vi "OLD Read Data File.vi"(0 "Filepath":path, 11 "Error In":errorcluster) -> (3 "Data":string[][](array[string]), 4 "Stats":string[][](array[string]), 6 "TestCfgCluster":T1, 8 "Serial Numbers":string[][](array[string]), 10 "TestParameters":string[][](array[string]), 15 "Error Out":errorcluster)   [LabVIEW 2013]
uses:
  TypeDef/TestCfgCluster.ctl
  TypeDef/Controller Names.ctl
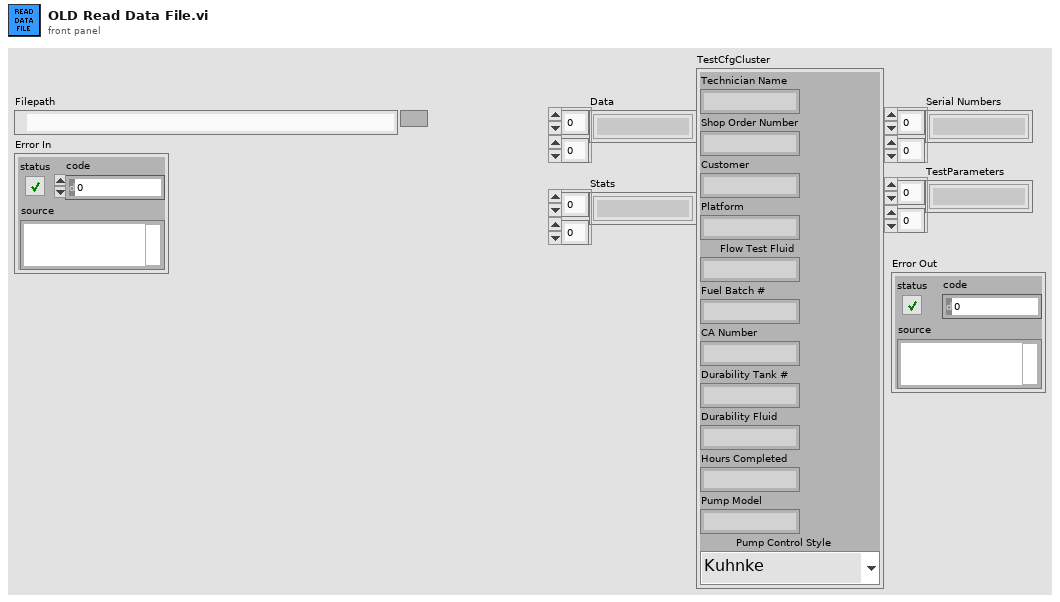
[diagram p1: front panel]
types:
  T1 = typedef "TestCfgCluster.ctl" = cluster{"Technician Name":string, "Shop Order Number":string, "Customer":string, "Platform":string, "Flow Test Fluid":string, "Fuel Batch #":string, "CA Number":string, "Durability Tank #":string, "Durability Fluid":string, "Hours Completed":string, "Pump Model":string, "Pump Control Style":T2}
  T2 = typedef "Controller Names.ctl" = enum16{"Kuhnke", "Conti", "Helbako", "TI PWM", "PSA", "Hella Gas", "Hella Diesel", "8 Comm", "10 Comm", "8 Comm Hella", "10 Comm Hella", "8 Comm Omron", "10 Comm Omron", "8 Comm Nissan", "10 Comm Nissan"}
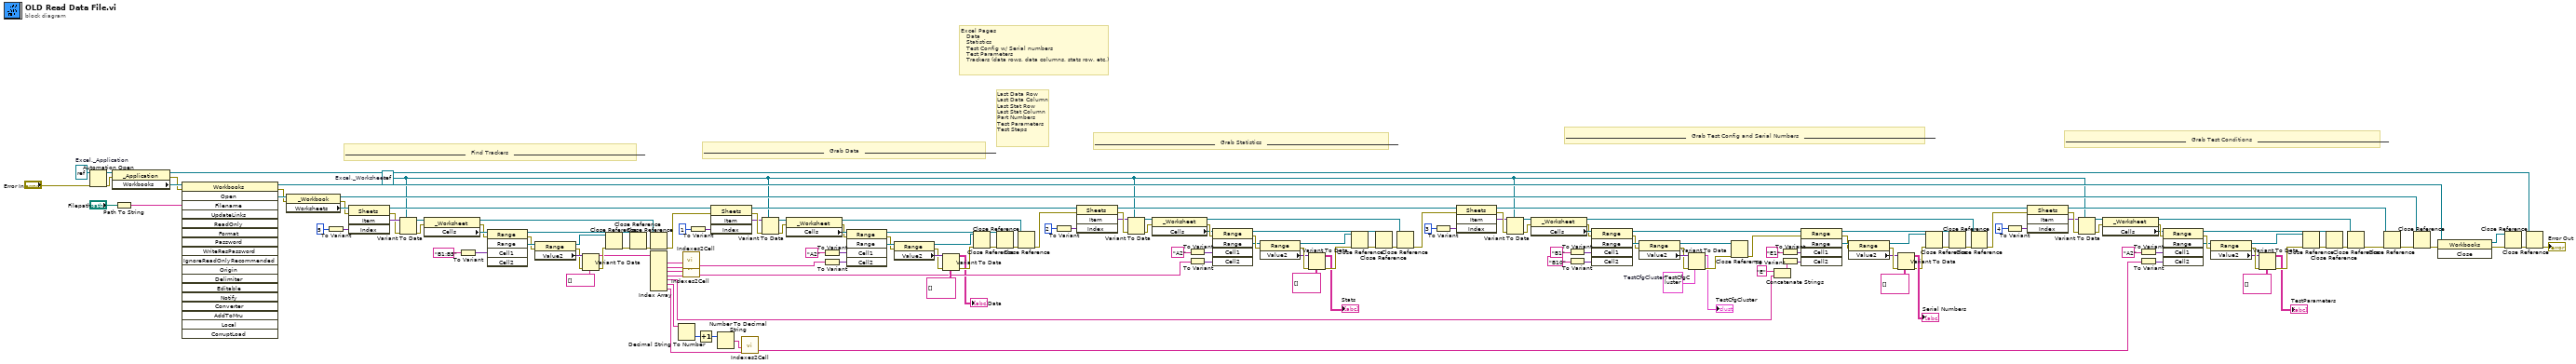
[diagram p0: block diagram]
diagram:
  w69 = T1 {"Technician Name"="", "Shop Order Number"="", "Customer"="", "Platform"="", "Flow Test Fluid"="", "Fuel Batch #"="", "CA Number"="", "Durability Tank #"="", "Durability Fluid"="", "Hours Completed"="", "Pump Model"="", "Pump Control Style"=enum."Kuhnke"}  # TestCfgCluster
  w12 = refnum<k7> refnum  # Excel._Worksheet
  w172 = refnum<k7> refnum  # Excel._Application
  # "___________________________________________   Grab Test Conditions   _______________________________________________"
  # "___________________________________________   Grab Test Config and Serial Numbers   _______________________________________________"
  # "___________________________________________   Grab Statistics   _______________________________________________"
  # "___________________________________________   Grab Data   _______________________________________________"
  # "___________________________________________   Find Trackers   _______________________________________________"
  # "Last Data Row\nLast Data Column\nLast Stat Row\nLast Stat Column\nPart Numbers\nTest Parameters\nTest Steps"
  # "Excel Pages\n   Data\n   Statistics\n   Test Config w/ Serial numbers\n   Test Parameters\n   Trackers (data rows, data columns, stats row, etc.)"
  n1 = Automation Open(error in (no error)="Error In", Automation Refnum=w172) -> (Automation Refnum=w173:refnum<k7>, error out=w174:errorcluster)  [unwired: 2 in]
  n2 = property class="_Application"(reference=w173, error in=w174) -> (reference out=w18:refnum<k7>, error out=w167:errorcluster, "Workbooks"=w175:refnum<k7>)
  n3 = Path To String(path="Filepath") -> (string=w170:string)
  n4 = invoke class="Workbooks" method="Open"(reference=w175, error in=w167, "Filename"=w170) -> (reference out=w22:refnum<k7>, error out=w168:errorcluster, "Open"=w171:refnum<k7>)  [unwired: 15 in, 15 out]
  n5 = property class="_Workbook"(reference=w171, error in=w168) -> (reference out=w23:refnum<k7>, error out=w147:errorcluster, "Worksheets"=w148:refnum<k7>)
  n6 = To Variant(anything=5) -> (Variant=w164:variant)
  n7 = invoke class="Sheets" method="Item"(reference=w148, error in=w147, "Index"=w164) -> (reference out=w143:refnum<k7>, error out=w162:errorcluster, "Item"=w163:variant)  [unwired: 1 in, 1 out]
  n8 = Variant To Data(error in=w162, type=w12, Variant=w163) -> (data=w161:refnum<k7>, error out=w154:errorcluster)
  n9 = property class="_Worksheet"(reference=w161, error in=w154) -> (reference out=w150:refnum<k7>, error out=w156:errorcluster, "Cells"=w160:refnum<k7>)
  n10 = To Variant(anything="B1:B5") -> (Variant=w157:variant)
  n11 = invoke class="Range" method="Range"(reference=w160, error in=w156, "Cell1"=w157) -> (reference out=w151:refnum<k7>, error out=w155:errorcluster, "Range"=w159:refnum<k7>)  [unwired: 2 in, 2 out]
  n12 = property class="Range"(reference=w159, error in=w155) -> (reference out=w153:refnum<k7>, error out=w134:errorcluster, "Value2"=w135:variant)
  n13 = Variant To Data(error in=w134, type=string[] [], Variant=w135) -> (data=w131:string[], error out=w133:errorcluster)
  n14 = Close Reference(reference=w153, error in (no error)=w133) -> (error out=w152:errorcluster)
  n15 = Close Reference(reference=w151, error in (no error)=w152) -> (error out=w149:errorcluster)
  n16 = Close Reference(reference=w150, error in (no error)=w149) -> (error out=w142:errorcluster)
  n17 = Index Array(array=w131) -> (element #1=w130:string, element #2=w129:string, element #3=w127:string, element #4=w126:string, element #5=w58:string, element #6=w29:string, element #7=w30:string)  [unwired: 7 in]
  n18 = Decimal String To Number(string=w29) -> (number=w32:i32)  [unwired: 2 in, 1 out]
  n19 = call "Indexes2Cell.vi"("RowIndex"=w130, "ColumnIndex"=w129) -> ("CellName"=w128:string)  [unwired: 5 in]
  n20 = call "Indexes2Cell.vi"("RowIndex"=w127, "ColumnIndex"=w126) -> ("CellName"=w92:string)  [unwired: 5 in]
  n21 = To Variant(anything=1) -> (Variant=w145:variant)
  n22 = Increment(x=w32) -> (x+1=w31:i32)
  n23 = invoke class="Sheets" method="Item"(reference=w143, error in=w142, "Index"=w145) -> (reference out=w94:refnum<k7>, error out=w141:errorcluster, "Item"=w6:variant)  [unwired: 1 in, 1 out]
  n24 = Number To Decimal String(number=w31) -> (decimal integer string=w28:string)  [unwired: 1 in]
  n25 = call "Indexes2Cell.vi"("RowIndex"=w28, "ColumnIndex"=w30) -> ("CellName"=w27:string)  [unwired: 5 in]
  n26 = Variant To Data(error in=w141, type=w12, Variant=w6) -> (data=w5:refnum<k7>, error out=w146:errorcluster)
  n27 = property class="_Worksheet"(reference=w5, error in=w146) -> (reference out=w115:refnum<k7>, error out=w121:errorcluster, "Cells"=w137:refnum<k7>)
  n28 = To Variant(anything="A2") -> (Variant=w140:variant)
  n29 = To Variant(anything=w128) -> (Variant=w136:variant)
  n30 = invoke class="Range" method="Range"(reference=w137, error in=w121, "Cell1"=w140, "Cell2"=w136) -> (reference out=w116:refnum<k7>, error out=w122:errorcluster, "Range"=w138:refnum<k7>)  [unwired: 1 in, 2 out]
  n31 = property class="Range"(reference=w138, error in=w122) -> (reference out=w117:refnum<k7>, error out=w123:errorcluster, "Value2"=w124:variant)
  n32 = Variant To Data(error in=w123, type=string[][] [], Variant=w124) -> (data=→"Data":string[][], error out=w120:errorcluster)
  n33 = Close Reference(reference=w117, error in (no error)=w120) -> (error out=w119:errorcluster)
  n34 = Close Reference(reference=w116, error in (no error)=w119) -> (error out=w118:errorcluster)
  n35 = Close Reference(reference=w115, error in (no error)=w118) -> (error out=w93:errorcluster)
  n36 = To Variant(anything=2) -> (Variant=w96:variant)
  n37 = invoke class="Sheets" method="Item"(reference=w94, error in=w93, "Index"=w96) -> (reference out=w71:refnum<k7>, error out=w98:errorcluster, "Item"=w7:variant)  [unwired: 1 in, 1 out]
  n38 = Variant To Data(error in=w98, type=w12, Variant=w7) -> (data=w8:refnum<k7>, error out=w95:errorcluster)
  n39 = property class="_Worksheet"(reference=w8, error in=w95) -> (reference out=w114:refnum<k7>, error out=w108:errorcluster, "Cells"=w102:refnum<k7>)
  n40 = To Variant(anything="A2") -> (Variant=w99:variant)
  n41 = To Variant(anything=w92) -> (Variant=w103:variant)
  n42 = invoke class="Range" method="Range"(reference=w102, error in=w108, "Cell1"=w99, "Cell2"=w103) -> (reference out=w113:refnum<k7>, error out=w107:errorcluster, "Range"=w101:refnum<k7>)  [unwired: 1 in, 2 out]
  n43 = property class="Range"(reference=w101, error in=w107) -> (reference out=w112:refnum<k7>, error out=w106:errorcluster, "Value2"=w105:variant)
  n44 = Variant To Data(error in=w106, type=string[][] [], Variant=w105) -> (data=→"Stats":string[][], error out=w109:errorcluster)
  n45 = Close Reference(reference=w112, error in (no error)=w109) -> (error out=w110:errorcluster)
  n46 = Close Reference(reference=w113, error in (no error)=w110) -> (error out=w111:errorcluster)
  n47 = Close Reference(reference=w114, error in (no error)=w111) -> (error out=w72:errorcluster)
  n48 = To Variant(anything=3) -> (Variant=w88:variant)
  n49 = invoke class="Sheets" method="Item"(reference=w71, error in=w72, "Index"=w88) -> (reference out=w16:refnum<k7>, error out=w86:errorcluster, "Item"=w10:variant)  [unwired: 1 in, 1 out]
  n50 = Variant To Data(error in=w86, type=w12, Variant=w10) -> (data=w9:refnum<k7>, error out=w89:errorcluster)
  n51 = property class="_Worksheet"(reference=w9, error in=w89) -> (reference out=w73:refnum<k7>, error out=w77:errorcluster, "Cells"=w82:refnum<k7>)
  n52 = To Variant(anything="B1") -> (Variant=w85:variant)
  n53 = To Variant(anything="B10") -> (Variant=w81:variant)
  n54 = invoke class="Range" method="Range"(reference=w82, error in=w77, "Cell1"=w85, "Cell2"=w81) -> (reference out=w3:refnum<k7>, error out=w78:errorcluster, "Range"=w83:refnum<k7>)  [unwired: 1 in, 2 out]
  n55 = property class="Range"(reference=w83, error in=w78) -> (reference out=w74:refnum<k7>, error out=w79:errorcluster, "Value2"=w80:variant)
  n56 = Variant To Data(error in=w79, type=w69, Variant=w80) -> (data=→"TestCfgCluster":T1, error out=w76:errorcluster)
  n57 = Close Reference(reference=w74, error in (no error)=w76) -> (error out=w61:errorcluster)
  n58 = Concatenate Strings("E", w58) -> (w59:string)
  n59 = To Variant(anything="E1") -> (Variant=w62:variant)
  n60 = To Variant(anything=w59) -> (Variant=w65:variant)
  n61 = invoke class="Range" method="Range"(reference=w3, error in=w61, "Cell1"=w62, "Cell2"=w65) -> (reference out=w2:refnum<k7>, error out=w4:errorcluster, "Range"=w64:refnum<k7>)  [unwired: 1 in, 2 out]
  n62 = property class="Range"(reference=w64, error in=w4) -> (reference out=w35:refnum<k7>, error out=w67:errorcluster, "Value2"=w66:variant)
  n63 = Variant To Data(error in=w67, type=string[][] [], Variant=w66) -> (data=→"Serial Numbers":string[][], error out=w36:errorcluster)
  n64 = Close Reference(reference=w35, error in (no error)=w36) -> (error out=w37:errorcluster)
  n65 = Close Reference(reference=w2, error in (no error)=w37) -> (error out=w75:errorcluster)
  n66 = Close Reference(reference=w73, error in (no error)=w75) -> (error out=w34:errorcluster)
  n67 = To Variant(anything=4) -> (Variant=w39:variant)
  n68 = invoke class="Sheets" method="Item"(reference=w16, error in=w34, "Index"=w39) -> (reference out=w13:refnum<k7>, error out=w41:errorcluster, "Item"=w17:variant)  [unwired: 1 in, 1 out]
  n69 = Variant To Data(error in=w41, type=w12, Variant=w17) -> (data=w11:refnum<k7>, error out=w38:errorcluster)
  n70 = property class="_Worksheet"(reference=w11, error in=w38) -> (reference out=w55:refnum<k7>, error out=w50:errorcluster, "Cells"=w45:refnum<k7>)
  n71 = To Variant(anything="A2") -> (Variant=w42:variant)
  n72 = To Variant(anything=w27) -> (Variant=w46:variant)
  n73 = invoke class="Range" method="Range"(reference=w45, error in=w50, "Cell1"=w42, "Cell2"=w46) -> (reference out=w54:refnum<k7>, error out=w49:errorcluster, "Range"=w44:refnum<k7>)  [unwired: 1 in, 2 out]
  n74 = property class="Range"(reference=w44, error in=w49) -> (reference out=w53:refnum<k7>, error out=w48:errorcluster, "Value2"=w47:variant)
  n75 = Variant To Data(error in=w48, type=string[][] [], Variant=w47) -> (data=→"TestParameters":string[][], error out=w51:errorcluster)
  n76 = Close Reference(reference=w53, error in (no error)=w51) -> (error out=w33:errorcluster)
  n77 = Close Reference(reference=w54, error in (no error)=w33) -> (error out=w52:errorcluster)
  n78 = Close Reference(reference=w55, error in (no error)=w52) -> (error out=w15:errorcluster)
  n79 = Close Reference(reference=w13, error in (no error)=w15) -> (error out=w14:errorcluster)
  n80 = Close Reference(reference=w23, error in (no error)=w14) -> (error out=w21:errorcluster)
  n81 = invoke class="Workbooks" method="Close"(reference=w22, error in=w21) -> (reference out=w20:refnum<k7>, error out=w19:errorcluster)  [unwired: 1 in, 1 out]
  n82 = Close Reference(reference=w20, error in (no error)=w19) -> (error out=w24:errorcluster)
  n83 = Close Reference(reference=w18, error in (no error)=w24) -> (error out=→"Error Out":errorcluster)
